vi "Initialize Attributes.vi"(8 "error in (no error)":errorcluster, 10 "Attribute Data":variant, 11 "CS++ControllerActor in":refnum<class "CS++ControllerActor.lvclass">) -> (0 "error out":errorcluster, 2 "Found?":bool, 3 "CS++ControllerActor out":refnum<class "CS++ControllerActor.lvclass">)   [LabVIEW 2014, in "CS++ControllerActor.lvlib" / "CS++ControllerActor.lvclass"]
doc: "Initialize object attribute.\n\nUnique resources should be allocated elsewhere!"
uses:
  CS++ControllerActor.lvclass
  Classes/CS++ProcessVariables/ProcessVariable/PV.lvclass
  CS++PVMonitor Messages/CS++PVUpdate Msg/CS++PVUpdate Msg.lvclass
  CS++BaseActor/CS++BaseActor.lvclass/CS++BaseActor.ctl
  Classes/CS++ProcessVariables/PVConnection/PVConnection.lvclass
  Classes/CS++ProcessVariables/ProcessVariable/PV.lvclass/PV.ctl
  CS++PVMonitor Messages/CS++PVUpdate Msg/CS++PVUpdate Msg.lvclass/CS++PVUpdate Msg.ctl
  CS++ControllerActor.lvclass/CS++ControllerActor.ctl
  Classes/CS++ProcessVariables/ProcessVariable/Write Name.vi
  Classes/CS++ProcessVariables/ProcessVariable/Write PV URL.vi
  CS++BaseActor/CS++BaseActor.lvclass
  Classes/CS++BaseClasses/Factory/CS++Factory.lvclass
  Libraries/Utilities/CS++Utilities.lvlib
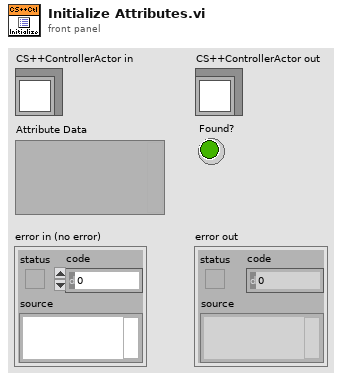
[diagram p1: front panel]
types:
  T1 = cluster{string, string, "CS++PVUpdate Msg out":refnum<class "CS++PVUpdate Msg.lvclass">, "CS++ProcessVariables.lvlib:PVConnection.lvclass":refnum<class "PVConnection.lvclass">}
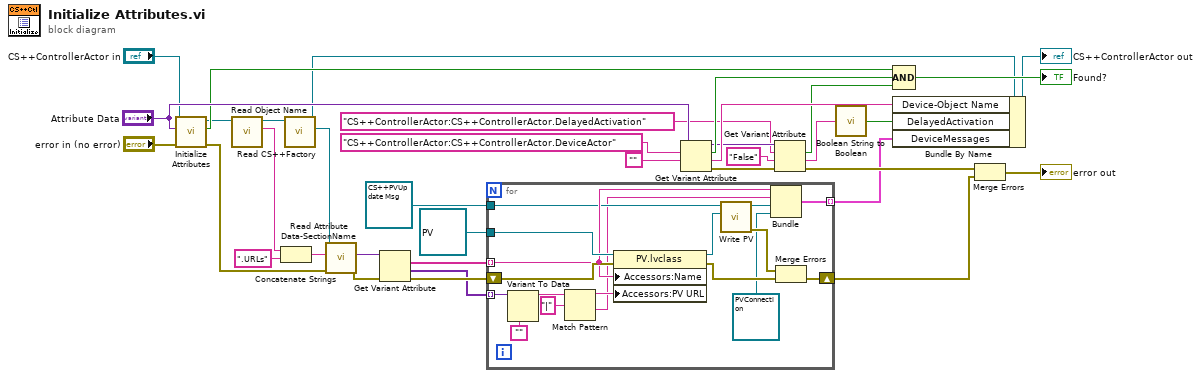
[diagram p0: block diagram]
diagram:
  n1 = call-parent "Initialize Attributes.vi"("error in (no error)"="error in (no error)", "Attribute Data"="Attribute Data", "CS++BaseActor in"="CS++ControllerActor in") -> ("error out"=w20:errorcluster, "Found?"=w28:bool, "CS++BaseActor out"=w25:refnum<class "CS++ControllerActor.lvclass">)  [unwired: 6 in]
  n2 = call "Read Object Name.vi"("CS++BaseActor in"=w25) -> ("Object Name"=w21:string, "CS++BaseActor out"=w26:refnum<class "CS++ControllerActor.lvclass">)  [unwired: 8 in, 1 out]
  n3 = Concatenate Strings(w21, ".URLs" ("string")) -> (w23:string)
  n4 = call "Read CS++Factory.vi"("CS++BaseActor in"=w26) -> ("CS++Factory"=w22:refnum<class "CS++Factory.lvclass">, "CS++BaseActor out"=w11:refnum<class "CS++ControllerActor.lvclass">)  [unwired: 8 in, 1 out]
  n5 = call-dynamic "Read Attribute Data-SectionName.vi"("error in (no error)"=w20, "Object Name"=w23, "CS++Factory in"=w22) -> ("error out"=w18:errorcluster, "Attribute Data"=w17:variant)  [unwired: 6 in, 1 out]
  n6 = Get Variant Attribute(Variant=w17, error in=w18) -> (names=w14:string[], values=w12:variant[], error out=w13:errorcluster)  [unwired: 2 in, 1 out]
  n7 = for {
    tunnel: refnum<class "PV.lvclass"> refnum ("CS++ProcessVariables.lvlib:PV.lvclass") -> [w53]
    shift-right: [w40] -> w16
    shift-left: w13 -> [w47]
    tunnel: w14 -> [w46] mode=indexing
    tunnel: w12 -> [w48] mode=indexing
    tunnel: [w45] -> w2 mode=indexing
    tunnel: refnum<class "CS++PVUpdate Msg.lvclass"> refnum ("CS++PVMonitor.lvlib:CS++PVUpdate Msg.lvclass") -> [w44]
    n8 = Variant To Data(type="", Variant=w48) -> (data=w49:string)  [unwired: 1 in, 1 out]
    n9 = Match Pattern(string=w49, regular expression="|" ("search string/char (-)")) -> (before substring=w52:string, after substring=w39:string)  [unwired: 1 in, 2 out]
    n10 = property class="PV.lvclass"(reference=w53, error in=w47, "Accessors:Name"=w46, "Accessors:PV URL"=w52) -> (reference out=w42:refnum<class "PV.lvclass">, error out=w38:errorcluster)
    n11 = call "Write PV.vi"("PV"=w42, "CS++PVUpdate Msg in"=w44) -> ("error out"=w41:errorcluster, "CS++PVUpdate Msg out"=w43:refnum<class "CS++PVUpdate Msg.lvclass">)  [unwired: 8 in]
    n12 = Bundle(w46, w39, "CS++PVUpdate Msg out"=w43, "CS++ProcessVariables.lvlib:PVConnection.lvclass"=refnum<class "PVConnection.lvclass"> refnum) -> (w45:T1)  [unwired: 1 in]
    n13 = Merge Errors(w41, w38) -> (w40:errorcluster)
  }
  n14 = Get Variant Attribute(Variant="Attribute Data", name="CS++ControllerActor:CS++ControllerActor.DeviceActor", default value (empty Variant)="") -> (duplicate Variant=w7:variant, found=w27:bool, value=w29:string, error out=w9:errorcluster)  [unwired: 1 in]
  n15 = Get Variant Attribute(Variant=w7, name="CS++ControllerActor:CS++ControllerActor.DelayedActivation", default value (empty Variant)="False", error in=w9) -> (found=w3:bool, value=w4:string, error out=w8:errorcluster)  [unwired: 1 out]
  n16 = call "Boolean String to Boolean.vi"("T/F String"=w4) -> ("Value"=w1:bool)
  n17 = Compound Arithmetic op=AND(w28, w27, w3) -> (→"Found?":bool)
  n18 = Bundle By Name(cluster=w11, "Device-Object Name"=w29, "DelayedActivation"=w1, "DeviceMessages"=w2) -> (→"CS++ControllerActor out":refnum<class "CS++ControllerActor.lvclass">)
  n19 = Merge Errors(w8, w16) -> (→"error out":errorcluster)
